vi "CLT_TestStateMach1.vi"(6 "Empty in":dbl=8.5, 8 "Full in":dbl=2.0, 9 "Level PV":dbl, 10 "Level SP":dbl, 11 "TEST State In":T2) -> (0 "Fill Cmd":bool, 1 "Drain Cmd":bool, 2 "SP Out":dbl, 3 "TEST State Out":T2, 4 "Ctl Sig":dbl)   [LabVIEW 2024]
doc: "The \"Run Test\" button selects between MANUAL adjustment of Set Point (SP) by the user or AUTO mode, where:\n1. Start, initial state drains until the tank is empty\n2. Filling, Auto set of SP to Max Fill Inches (or recipie)\n3. FULL Pause when full\n4. Draining Auto set of SP to 0 (or recipie)\n5. EMPTY Paue when empty\n6. Done SP set to 0."
uses:
  Control Definitions/Global 2.vi
  Control Definitions/Def TestState.ctl
  Control Definitions/Def PumpCtlRefs.ctl
panel:
  in  "cluster":T1
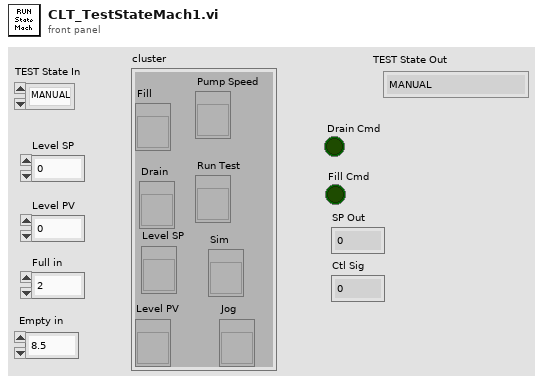
[diagram p1: front panel]
types:
  T1 = typedef "Def PumpCtlRefs.ctl" = cluster{"Fill ":refnum<vi>, "Drain":refnum<vi>, "Level PV":refnum<vi>, "Pump Speed":refnum<vi>, "Run Test":refnum<vi>, "Sim":refnum<vi>, "Jog":refnum<vi>, "Level SP":refnum<vi>}
  T2 = typedef "Def TestState.ctl" = enum16{"MANUAL", "Start", "Pre-Fill", "Pre-Drain", "Start-Record", "Load Fill Spec", "Filling Lo", "BinSearch Fill", "Record Fill", "Load Drain Spec", "Draining Hi", "BinSearch Drain", "Record Drain", "Empty", "Done"}
  T3 = enum16{"MANUAL", "Start", "Filling", "FULL", "Draining", "EMPTY", "Done"}
  T4 = enum16{"MANUAL", "Start", "Pre-Fill", "Pre-Drain", "Start-Record", "Filling", "FULL", "Draining", "EMPTY", "Done"}
  T5 = typedef "Def TestState.ctl" = enum16{"MANUAL", "Start", "Pre-Fill", "Pre-Drain", "Start-Record", "Filling", "FULL", "Draining", "EMPTY", "Done"}
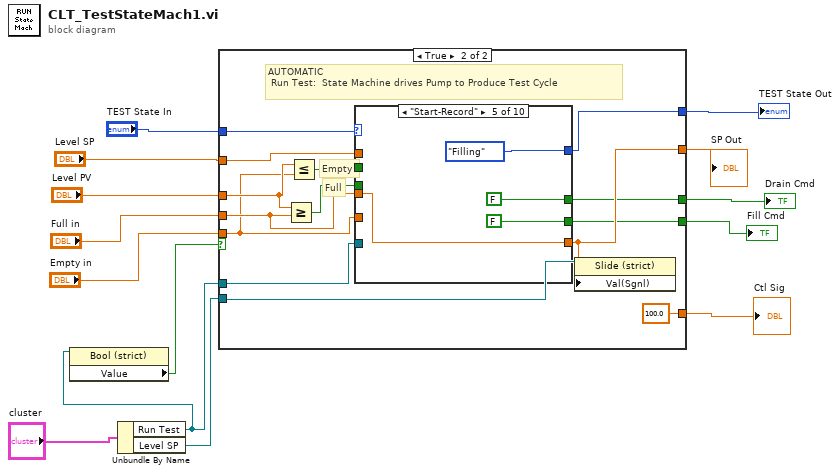
[diagram p0: block diagram]
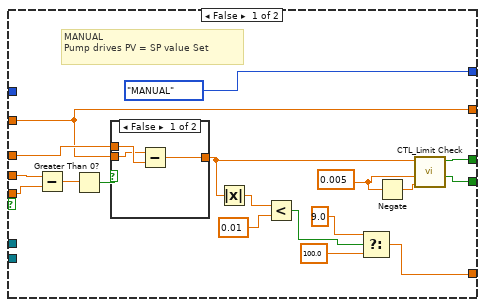
[diagram p2: hidden frame]
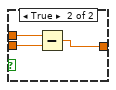
[diagram p3: hidden frame]
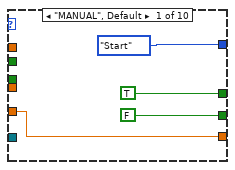
[diagram p4: hidden frame]
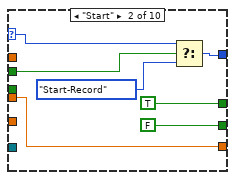
[diagram p5: hidden frame]
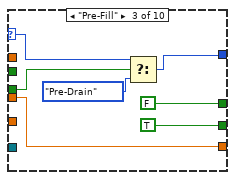
[diagram p6: hidden frame]
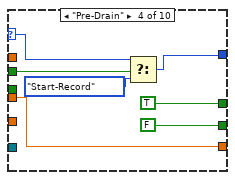
[diagram p7: hidden frame]
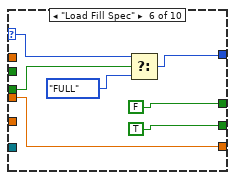
[diagram p8: hidden frame]
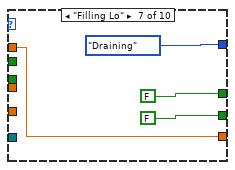
[diagram p9: hidden frame]
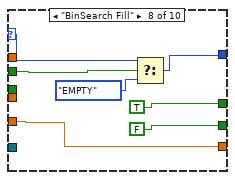
[diagram p10: hidden frame]
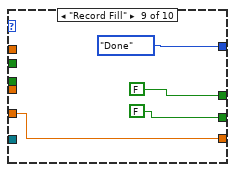
[diagram p11: hidden frame]
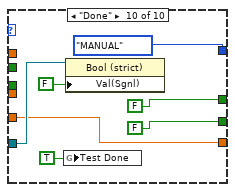
[diagram p12: hidden frame]
diagram:
  n1 = Unbundle By Name("cluster") -> ("Run Test"=w11:refnum<vi>, "Level SP"=w10:refnum<vi>)
  n2 = property class="Bool (strict)"(reference=w11) -> ("Value"=w4:bool)  [unwired: 1 in, 2 out]
  n3 = case shown="True" w4 {
    tunnel: "Level SP" -> [w27 w48]
    tunnel: "TEST State In" -> [_ w39]
    tunnel: "Level PV" -> [w28 w42]
    tunnel: [T3."MANUAL" ("TEST STATUS In in") w51] -> w2
    tunnel: "Full in" -> [w25 w52]
    tunnel: "Empty in" -> [w24 w41]
    tunnel: w11 -> [_ w47]
    tunnel: w10 -> [_ w46]
    tunnel: [w27 w45] -> w9
    tunnel: [w26 w44] -> w8
    tunnel: [w30 w43] -> w7
    tunnel: [w18 100.0] -> w3
    frame False {
      w29 = 0.005 ("Pos Limit")
      # "MANUAL \nPump drives PV = SP value Set"
      n4 = Subtract(x=w25, y=w24) -> (x-y=w23:dbl)
      n5 = Greater Than 0?(x=w23) -> (x > 0?=w22:bool)
      n6 = case shown="False" w22 {
        tunnel: [w33 w38] -> w21
        tunnel: w28 -> [w35 w37]
        tunnel: w27 -> [w34 w36]
        frame False {
          n7 = Subtract(x=w34, y=w35) -> (x-y=w33:dbl)
        }
        frame True {
          n8 = Subtract(x=w37, y=w36) -> (x-y=w38:dbl)
        }
      }
      n9 = Absolute Value(x=w21) -> (abs(x)=w20:dbl)
      n10 = Less?(x=w20, y=0.01) -> (x < y?=w15:bool)
      n11 = Select(t=9.0, s=w15, f=100.0) -> (s? t:f=w18:dbl)
      n12 = Negate(x=w29) -> (-x=w31:dbl)
      n13 = call "CTL_Limit Check.vi"("Neg Limit"=w31, "Pos Limit"=w29, "X"=w21) -> ("X< Neg"=w30:bool, "X>Pos"=w26:bool)  [unwired: 6 in, 1 out]
    }
    frame True {
      # "Full"
      # "Empty"
      # "AUTOMATIC\n Run Test:  State Machine drives Pump to Produce Test Cycle"
      n14 = Greater Or Equal?(x=w42, y=w52) -> (x >= y?=w49:bool)
      n15 = Less Or Equal?(x=w42, y=w41) -> (x <= y?=w50:bool)
      n16 = case shown="\"Start-Record\"" w39 {
        selector: w39 -> [_ w63 w70 w77 _ w86 _ w98 _ _]
        tunnel: w52 -> [_ w59 w66 w73 w79 w83 _ _ _ _]
        tunnel: [w54 w59 w66 w73 w79 w83 w90 w96 w101 w106] -> w45
        tunnel: [Def_TestState."Start" ("TEST State Out") w62 w69 w76 Def_TestState."Filling" ("TEST State Out") w88 Def_TestState."Draining" ("TEST State Out") w99 Def_TestState."Done" ("TEST State Out") Def_TestState."MANUAL" ("TEST State Out")] -> w51
        tunnel: w50 -> [_ w58 _ w72 _ _ _ w97 _ _]
        tunnel: w49 -> [_ _ w65 _ _ w87 _ _ _ _]
        tunnel: w41 -> [w54 _ _ _ _ _ _ w96 w101 w106]
        tunnel: w48 -> [_ _ _ _ _ _ w90 _ _ _]
        tunnel: w47 -> [_ _ _ _ _ _ _ _ _ w110]
        tunnel: [TRUE TRUE FALSE TRUE FALSE FALSE FALSE TRUE FALSE FALSE] -> w44
        tunnel: [FALSE FALSE TRUE FALSE FALSE TRUE FALSE FALSE FALSE FALSE] -> w43
        frame "MANUAL", Default {
        }
        frame "Start" {
          n17 = Select(t=w63, s=w58, f=Def_TestState."Start-Record" ("s? t:f")) -> (s? t:f=w62:T2)
        }
        frame "Pre-Fill" {
          n18 = Select(t=w70, s=w65, f=T4."Pre-Drain" ("TEST STATUS In")) -> (s? t:f=w69:u16)
        }
        frame "Pre-Drain" {
          n19 = Select(t=w77, s=w72, f=T4."Start-Record" ("TEST STATUS In")) -> (s? t:f=w76:u16)
        }
        frame "Start-Record" {
        }
        frame "Load Fill Spec" {
          n20 = Select(t=w86, s=w87, f=Def_TestState."FULL" ("TEST State Out")) -> (s? t:f=w88:u16)
        }
        frame "Filling Lo" {
        }
        frame "BinSearch Fill" {
          n21 = Select(t=w98, s=w97, f=Def_TestState."EMPTY" ("TEST State Out")) -> (s? t:f=w99:u16)
        }
        frame "Record Fill" {
        }
        frame "Done" {
          n22 = global write "Global 2.vi" "Test Done"(TRUE ("Test Done")) -> ()
          n23 = property class="Bool (strict)"(reference=w110, "Val(Sgnl)"=FALSE ("Value (Signaling)")) -> ()  [unwired: 1 in, 2 out]
        }
      }
      n24 = property class="Slide (strict)"(reference=w46, "Val(Sgnl)"=w45) -> ()  [unwired: 1 in, 2 out]
    }
  }
  "SP Out" <- w9
  "Fill Cmd" <- w7
  "Drain Cmd" <- w8
  "Ctl Sig" <- w3
  "TEST State Out" <- w2
